vi "Select 3 mA Chan.vi"(1 "Output Level (1.0 mA)":dbl) -> (0 "Chan Array":T1(array[cluster]))   [LabVIEW 2018, in "Agilent U2722.lvlib"]
uses:
  U2722 LabVIEW Instr Driver and Examples/Agilent U2722.lvlib
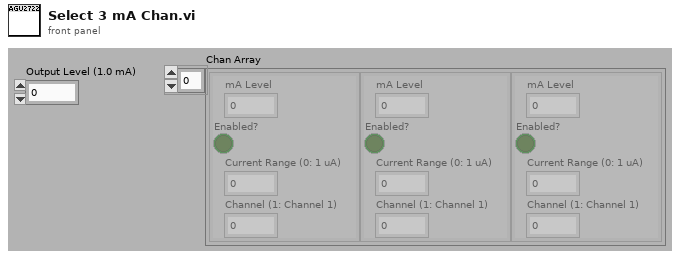
[diagram p1: front panel]
types:
  T1 = cluster{"mA Level":dbl, "Enabled?":bool, "Current Range (0: 1 uA)":u16, "Channel (1: Channel 1)":u16}[]
  T2 = cluster{"mA Level":dbl, "Enabled?":bool, "Current Range (0: 1 uA)":u16, "Channel (1: Channel 1)":u16}
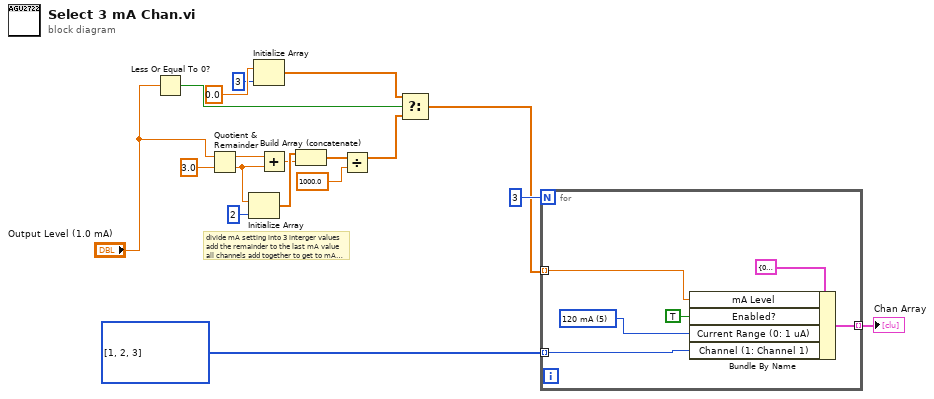
[diagram p0: block diagram]
diagram:
  w18 = u16[] [1, 2, 3] items=["Channel 1"=1, "Channel 2"=2, "Channel 3"=3] ("Array")
  # "divide mA setting into 3 interger values\nadd the remainder to the last mA value\nall channels add together to get to mA setting"
  n1 = Less Or Equal To 0?(x="Output Level (1.0 mA)") -> (x <= 0?=w16:bool)
  n2 = Quotient & Remainder(x="Output Level (1.0 mA)", y=3.0) -> (x-y*floor(x/y)=w10:dbl, floor(x/y)=w9:dbl)
  n3 = Initialize Array(w9, 2 ("dimension size")) -> (w11:dbl[])
  n4 = Initialize Array(0.0 ("t"), 3 ("dimension size")) -> (w1:dbl[])
  n5 = Add(x=w10, y=w9) -> (x+y=w8:dbl)
  n6 = Build Array (concatenate)(w11, w8) -> (w7:dbl[])
  n7 = Divide(x=w7, y=1000.0) -> (x/y=w5:dbl[])
  n8 = Select(t=w1, s=w16, f=w5) -> (s? t:f=w14:dbl[])
  n9 = for {
    N: 3 -> [_]
    tunnel: [w23] -> w17 mode=indexing
    tunnel: w18 -> [w22] mode=indexing
    tunnel: w14 -> [w21] mode=indexing
    w19 = u16 5 items=["1 uA", "10 uA", "100 uA", "1 mA", "10 mA", "120 mA"] ("Current Range (0: 1 uA)")
    n10 = Bundle By Name(cluster=T2 {"mA Level"=0.0, "Enabled?"=FALSE, "Current Range (0: 1 uA)"=0, "Channel (1: Channel 1)"=1}, "mA Level"=w21, "Enabled?"=TRUE, "Current Range (0: 1 uA)"=w19, "Channel (1: Channel 1)"=w22) -> (w23:T2)
  }
  "Chan Array" <- w17
